vi "Start Sync.vi"(8 "error in (no error)":errorcluster, 11 "gRPC Server in":refnum<class "GreeterService.lvclass">) -> (0 "error out":errorcluster, 3 "gRPC Server out":refnum<class "GreeterService.lvclass">)   [LabVIEW 2019, in "Generated_server.lvlib" / "GreeterService.lvclass"]
uses:
  GreeterService.lvclass
  GreeterService.lvclass/GreeterService.ctl
  RPC Messages/Greeter_res.ctl
  RPC Messages/Greeter_res_res_oneof/Greeter_res_res_oneof.lvclass
  RPC Messages/Greeter_req_req_oneof/Greeter_req_req_oneof.lvclass/Greeter_req_req_oneof.ctl
  RPC Messages/Greeter_res_res_oneof/Greeter_res_res_oneof.lvclass/Greeter_res_res_oneof.ctl
  Generated_server.lvlib
  RPC Messages/Greeter_req_req_oneof/Greeter_req_req_oneof.lvclass
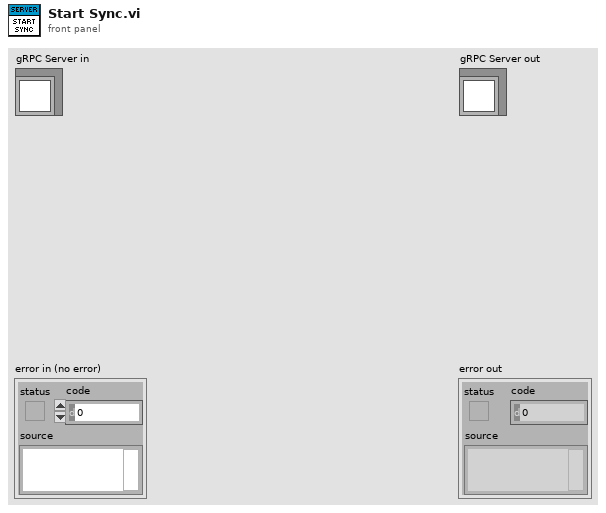
[diagram p1: front panel]
types:
  T1 = typedef "Generated_server.lvlib/Greeter_res.ctl" = cluster{"res_latitude":i32, "Greeter_res_res_oneof":refnum<class "Greeter_res_res_oneof.lvclass">}
  T2 = typedef "Generated_server.lvlib/GreeterService.lvclass/Server Internal UEs.ctl" = cluster{"GreeterService GetFeature Internal UE":refnum<user-event>}
  T3 = typedef "Generated_server.lvlib/GreeterService.lvclass/Server gRPC UEs.ctl" = cluster{"GreeterService GetFeature gRPC UE":refnum<user-event>}
  T4 = typedef "grpc-lvsupport-release.lvlib/grpcId.ctl" = u64
  T5 = typedef "Generated_server.lvlib/Greeter_req.ctl" = cluster{"req_latitude":i32, "Greeter_req_req_oneof":refnum<class "Greeter_req_req_oneof.lvclass">}
  T6 = typedef "grpc-lvsupport.lvlib/grpcId.ctl" = u64
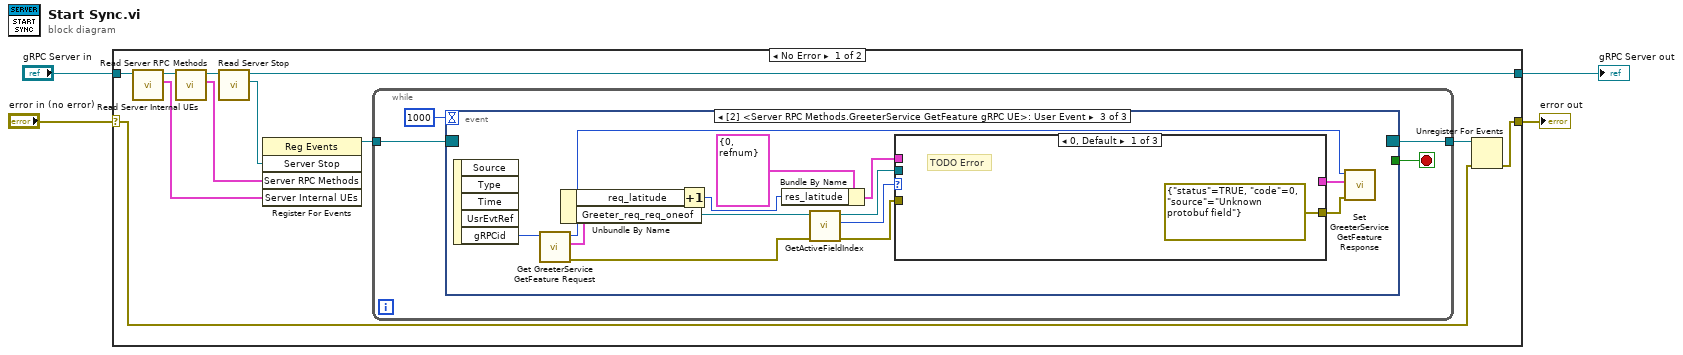
[diagram p0: block diagram]
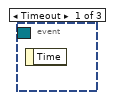
[diagram p2: hidden frame]
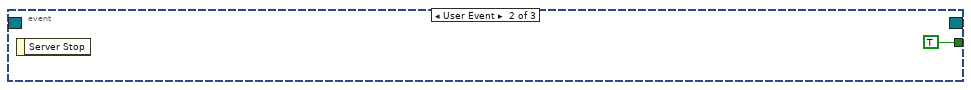
[diagram p3: hidden frame]
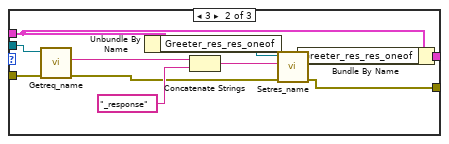
[diagram p4: hidden frame]
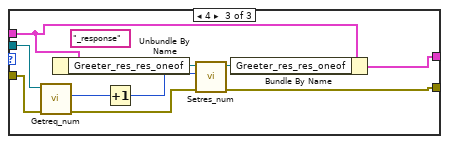
[diagram p5: hidden frame]
diagram:
  n1 = case shown="No Error" "error in (no error)" {
    selector: "error in (no error)" -> [w9 w58]
    tunnel: [w8 w58] -> w3
    tunnel: [w6 w57] -> w1
    tunnel: "gRPC Server in" -> [w15 w57]
    frame No Error {
      n2 = call "Read Server Internal UEs.vi"("SignalGeneratorService in"=w15) -> ("Server Internal UEs"=w13:T2, "SignalGeneratorService out"=w14:refnum<class "GreeterService.lvclass">)  [unwired: 8 in, 1 out]
      n3 = call "Read Server RPC Methods.vi"("SignalGeneratorService in"=w14) -> ("Server RPC Methods"=w7:T3, "SignalGeneratorService out"=w12:refnum<class "GreeterService.lvclass">)  [unwired: 8 in, 1 out]
      n4 = call-dynamic "Read Server Stop.vi"("iService in"=w12) -> ("Server Stop"=w5:refnum<user-event>, "iService out"=w6:refnum<class "GreeterService.lvclass">)  [unwired: 8 in, 1 out]
      n5 = register-events(w5, w7, w13) -> (reference out=w11:refnum<event-registration>)  [unwired: 2 in, 1 out]
      n6 = while {
        tunnel: w11 -> [w19]
        tunnel: [w17] -> w10
        stop <- w18 stop-if-true
        n7 = event "RPC Methods Event Structure" shown="[2] <Server RPC Methods.GreeterService GetFeature gRPC UE>: User Event" {
          selector: w19 -> [_ _ _]
          dyn-events: [_ _ _] -> w17
          timeout: 1000 -> [_ _ _]
          tunnel: [_ TRUE _] -> w18
          event Timeout {
            n8 = event-data() -> ()  [unwired: 1 in, 1 out]
          }
          event User Event {
            n9 = event-data() -> ()  [unwired: 1 in, 1 out]
          }
          event User Event {
            n10 = event-data() -> ("gRPCid"=w34:T4)  [unwired: 1 in, 4 out]
            n11 = call "Get GreeterService GetFeature Request.vi"("gRPCid in"=w34) -> ("error out"=w27:errorcluster, "Message Data"=w32:T5, "gRPCid out"=w33:T6)  [unwired: 8 in]
            n12 = Unbundle By Name(w32) -> ("req_latitude"=w30:i32, "Greeter_req_req_oneof"=w28:refnum<class "Greeter_req_req_oneof.lvclass">)
            n13 = Increment(x=w30) -> (x+1=w29:i32)
            n14 = Bundle By Name(cluster=T1 {"res_latitude"=0, "Greeter_res_res_oneof"=refnum} ("Message Data"), "res_latitude"=w29) -> (w23:T1)
            n15 = call "GetActiveFieldIndex.vi"("error in (no error)"=w27, "OneOfTemplate in"=w28) -> ("error out"=w24:errorcluster, "Active Field Index"=w26:i32, "OneOfTemplate out"=w25:refnum<class "Greeter_req_req_oneof.lvclass">)  [unwired: 7 in]
            n16 = case shown="0, Default" w26 {
              tunnel: w25 -> [_ w46 w56]
              tunnel: w24 -> [_ w45 w55]
              tunnel: w23 -> [_ w43 w53]
              tunnel: [_ w38 w51] -> w22
              tunnel: [errorcluster {"status"=TRUE, "code"=0, "source"="Unknown protobuf field"} ("error out") w36 w47] -> w21
              frame 0, Default {
                # "TODO Error"
              }
              frame 3 {
                n17 = call "Getreq_name.vi"("error in (no error)"=w45, "OneOfTemplate in"=w46) -> ("error out"=w37:errorcluster, "Get_Val"=w40:string)  [unwired: 7 in, 1 out]
                n18 = Unbundle By Name(w43) -> ("Greeter_res_res_oneof"=w42:refnum<class "Greeter_res_res_oneof.lvclass">)
                n19 = Concatenate Strings(w40, "_response") -> (w39:string)
                n20 = call "Setres_name.vi"("error in (no error)"=w37, "Set_Val"=w39, "OneOfTemplate in"=w42) -> ("error out"=w36:errorcluster, "OneOfTemplate out"=w44:refnum<class "Greeter_res_res_oneof.lvclass">)  [unwired: 7 in]
                n21 = Bundle By Name(cluster=w43, "Greeter_res_res_oneof"=w44) -> (w38:T1)
              }
              frame 4 {
                (unwired) "_response"
                n22 = call "Getreq_num.vi"("error in (no error)"=w55, "OneOfTemplate in"=w56) -> ("error out"=w48:errorcluster, "Get_Val"=w50:i32)  [unwired: 7 in, 1 out]
                n23 = Unbundle By Name(w53) -> ("Greeter_res_res_oneof"=w52:refnum<class "Greeter_res_res_oneof.lvclass">)
                n24 = Increment(x=w50) -> (x+1=w49:i32)
                n25 = call "Setres_num.vi"("error in (no error)"=w48, "Set_Val"=w49, "OneOfTemplate in"=w52) -> ("error out"=w47:errorcluster, "OneOfTemplate out"=w54:refnum<class "Greeter_res_res_oneof.lvclass">)  [unwired: 7 in]
                n26 = Bundle By Name(cluster=w53, "Greeter_res_res_oneof"=w54) -> (w51:T1)
              }
            }
            n27 = call "Set GreeterService GetFeature Response.vi"("error in (no error)"=w21, "Message Data"=w22, "gRPCid in"=w33) -> ()  [unwired: 8 in, 1 out]
          }
        }
      }
      n28 = Unregister For Events(event registration refnum=w10, error in=w9) -> (error out=w8:errorcluster)
    }
    frame Error {
    }
  }
  "error out" <- w3
  "gRPC Server out" <- w1
